vi "CheckIfTerminalConnected.vi"(8 "Error In":errorcluster, 11 "ControlTerminal":refnum<vi>) -> (0 "Error Out":errorcluster, 2 "Wire terminal references":refnum<vi>[](array[refnum]), 3 "Terminal is connected to other(s)?":bool)   [LabVIEW 2017, in "ErrorStructureDrawer.lvlib"]
doc: "Checks if a terminal is connected to any other terminal(s).\n\nIf connected, also returns an array of references to the connecting wire's terminal(s)."
uses:
  ErrorStructureDrawer.lvlib
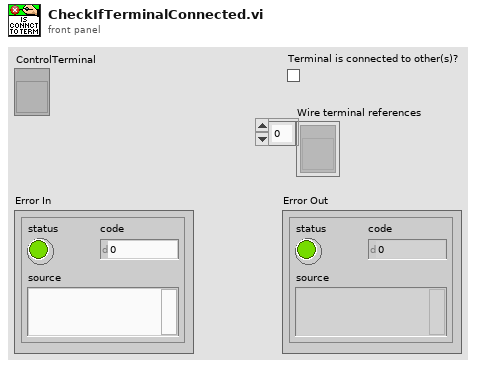
[diagram p1: front panel]
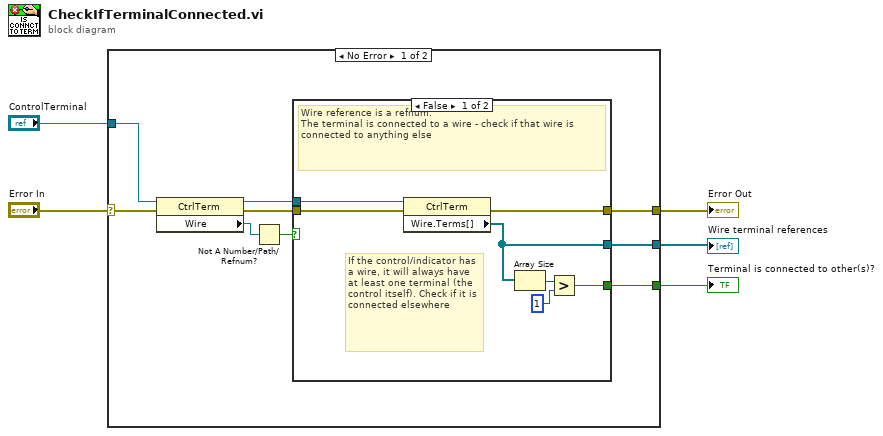
[diagram p0: block diagram]
diagram:
  n1 = case shown="No Error" "Error In" {
    selector: "Error In" -> [w9 w23]
    tunnel: "ControlTerminal" -> [w14 _]
    tunnel: [w10 _] -> w4
    tunnel: [w8 w23] -> w2
    tunnel: [w7 _] -> w1
    frame No Error {
      n2 = property class="CtrlTerm"(reference=w14, error in=w9) -> (reference out=w6:refnum<vi>, error out=w12:errorcluster, "Wire"=w13:refnum<vi>)
      n3 = Not A Number/Path/Refnum?(number/path/refnum=w13) -> (NaN/Path/Refnum?=w11:bool)
      n4 = case shown="False" w11 {
        tunnel: w12 -> [w20 w22]
        tunnel: [w18 _] -> w10
        tunnel: [w17 w22] -> w8
        tunnel: [w16 _] -> w7
        tunnel: w6 -> [w15 _]
        frame False {
          # "If the control/indicator has a wire, it will always have at least one terminal (the control itself). Check if it is connected elsewhere"
          # "Wire reference is a refnum:\nThe terminal is connected to a wire - check if that wire is connected to anything else"
          n5 = property class="CtrlTerm"(reference=w15, error in=w20) -> (error out=w17:errorcluster, "Wire.Terms[]"=w16:refnum<vi>[])  [unwired: 1 out]
          n6 = Array Size(array=w16) -> (size(s)=w21:i32)
          n7 = Greater?(x=w21, y=1) -> (0:w18:bool)
        }
        frame True {
          # "Wire reference is not-a-refnum:\nThe terminal isn't connected to a wire, so it isn't connected to anything else"
        }
      }
    }
    frame Error {
    }
  }
  "Terminal is connected to other(s)?" <- w4
  "Error Out" <- w2
  "Wire terminal references" <- w1
